vi "IStageMoveBack.vi"(0 "PRIORLib.IStageIn":refnum<k7>, 1 "Distance":dbl=1000.0) -> (2 "PRIORLib.IStageOut":refnum<k7>, 3 "error out":errorcluster, 4 "MoveBack":i32)   [LabVIEW 2011]
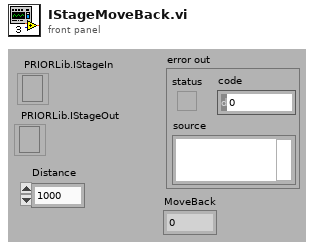
[diagram p1: front panel]
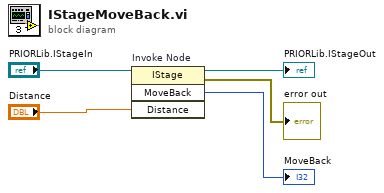
[diagram p0: block diagram]
diagram:
  n1 = invoke on="Invoke Node" class="IStage" method="MoveBack"(reference="PRIORLib.IStageIn", "Distance"="Distance") -> (reference out=→"PRIORLib.IStageOut":refnum<k7>, error out=→"error out":errorcluster, "MoveBack"=→"MoveBack":i32)  [unwired: 2 in, 1 out]
